vi "Set File Paths.vi"(9 "Log File Path":path, 10 "CID File Path":path, 11 "SCADA in":refnum<class "SCADA.lvclass">) -> (3 "SCADA out":refnum<class "SCADA.lvclass">)   [LabVIEW 2015, in "SCADA Core.lvlib" / "SCADA.lvclass"]
uses:
  SCADA.lvclass
  SCADA.lvclass/SCADA.ctl
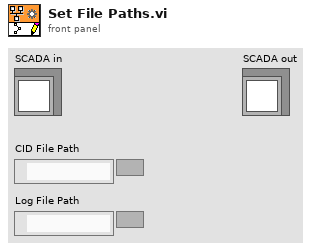
[diagram p1: front panel]
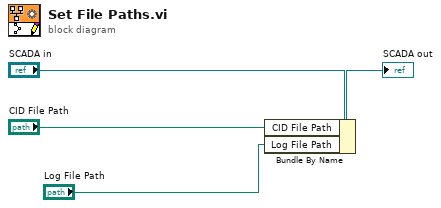
[diagram p0: block diagram]
diagram:
  n1 = Bundle By Name(cluster="SCADA in", "CID File Path"="CID File Path", "Log File Path"="Log File Path") -> (→"SCADA out":refnum<class "SCADA.lvclass">)
